vi "Set Column Type.vi"(8 "error in (no error)":errorcluster, 10 "Column Type":T1, 11 "Basic Column Configuration in":refnum<class "Basic Column Configuration.lvclass">) -> (0 "error out":errorcluster, 3 "Basic Column Configuration out":refnum<class "Basic Column Configuration.lvclass">)   [LabVIEW 2020, in "Basic Columns.lvlib" / "Basic Column Configuration.lvclass"]
uses:
  Basic Column Configuration.lvclass
  Database Interfaces/Database data type.ctl
  Basic Column Configuration.lvclass/Basic Column Configuration.ctl
  Database Interfaces.lvlib
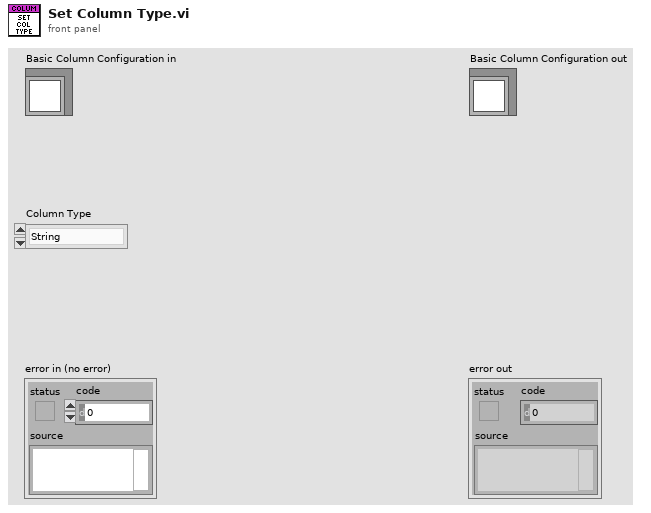
[diagram p1: front panel]
types:
  T1 = typedef "Database Interfaces.lvlib/Database data type.ctl" = enum16{"String", "Long (I32)", "Single (SGL)", "Double (DBL)", "Date/Time", "Binary"}
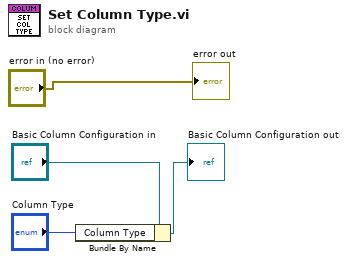
[diagram p0: block diagram]
diagram:
  n1 = Bundle By Name(cluster="Basic Column Configuration in", "Column Type"="Column Type") -> (→"Basic Column Configuration out":refnum<class "Basic Column Configuration.lvclass">)
  "error out" <- "error in (no error)"
